vi "Camera_Read and Save Settings.vi"(8 "Error":errorcluster, 10 "CameraDevRef":T7, 11 "Camera Address":string) -> (0 "Error Out":errorcluster, 1 "Output Cluster Out":T1, 2 "Camera Settings Out":T2 {"Saturation" min=0 max=100 step=1; "Sharpness" min=0 max=100 step=1; "Brightness" min=0 max=100 step=1; "Exposure (%)" min=0.0 max=100.0 step=1.0}, 3 "CameraDevRef Out":T7)   [LabVIEW 2017, in "VisionSystem.lvlib"]
uses:
  VisionSystem.lvlib
  <vilib>/Rock Robotics/WPI/Camera/WPI_CameraDevRef.ctl
  TypeDefs/Cluster_Camera Settings.ctl
  <vilib>/Rock Robotics/WPI/Camera/WPI_CameraImageSize.ctl
  <vilib>/Rock Robotics/WPI/Camera/WPI_CameraFrameRate.ctl
  <vilib>/Rock Robotics/WPI/Camera/WPI_CameraWhite Balance Values.ctl
  <vilib>/Rock Robotics/WPI/Camera/WPI_CameraExposure Values.ctl
  <vilib>/Rock Robotics/WPI/Camera/WPI_CameraSettings Control.ctl
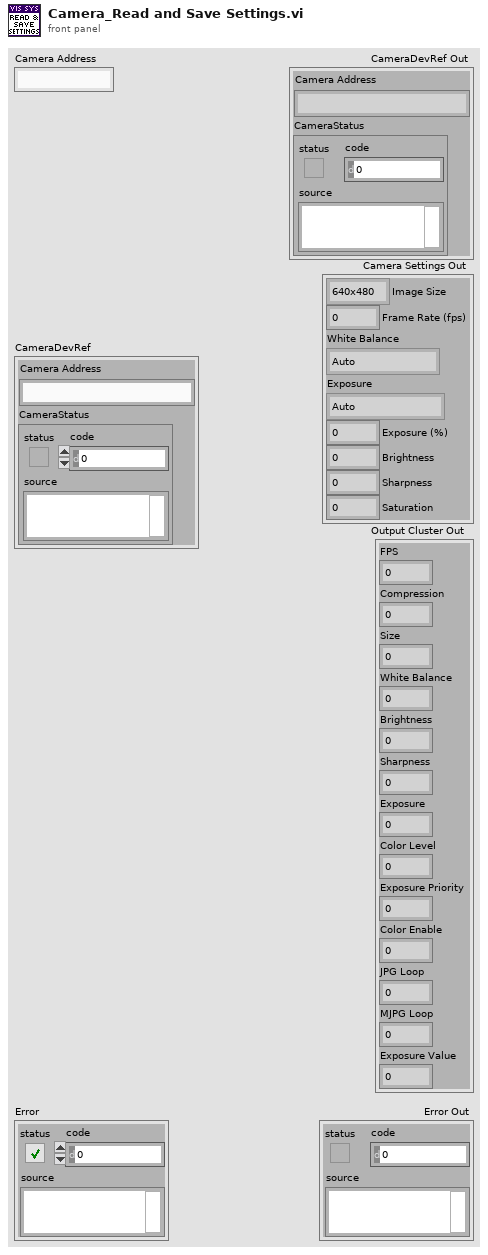
[diagram p1: front panel]
types:
  T1 = typedef "WPI_CameraSettings Control.ctl" = cluster{"FPS":i32, "Compression":i32, "Size":i32, "White Balance":i32, "Brightness":i32, "Sharpness":i32, "Exposure":i32, "Color Level":i32, "Exposure Priority":i32, "Color Enable":i32, "JPG Loop":i32, "MJPG Loop":i32, "Exposure Value":i32}
  T2 = typedef "Cluster_Camera Settings.ctl" = cluster{"Image Size":T3, "Frame Rate (fps)":T4, "White Balance":T5, "Exposure":T6, "Exposure (%)":dbl, "Brightness":i32, "Sharpness":i32, "Saturation":i32}
  T3 = typedef "WPI_CameraImageSize.ctl" = enum16{"640x480", "320x240", "160x120", "Custom"}
  T4 = typedef "WPI_CameraFrameRate.ctl" = u32
  T5 = typedef "WPI_CameraWhite Balance Values.ctl" = enum16{"Auto", "Fixed indoor", "Fixed outdoor 1", "Fixed outdoor 2", "Fixed fluorescent 1", "Fixed fluorescent 2", "Hold current", "Custom"}
  T6 = typedef "WPI_CameraExposure Values.ctl" = enum16{"Auto", "Flicker-free 50 Hz", "Flicker-free 60 Hz", "Hold current", "Custom"}
  T7 = typedef "WPI_CameraDevRef.ctl" = cluster{"Camera Address":string, "CameraStatus":errorcluster}
  T8 = typedef "WPI_CameraExposure Priority Values.ctl" = enum16{"None", "Prioritize frame rate", "Prioritize image quality"}
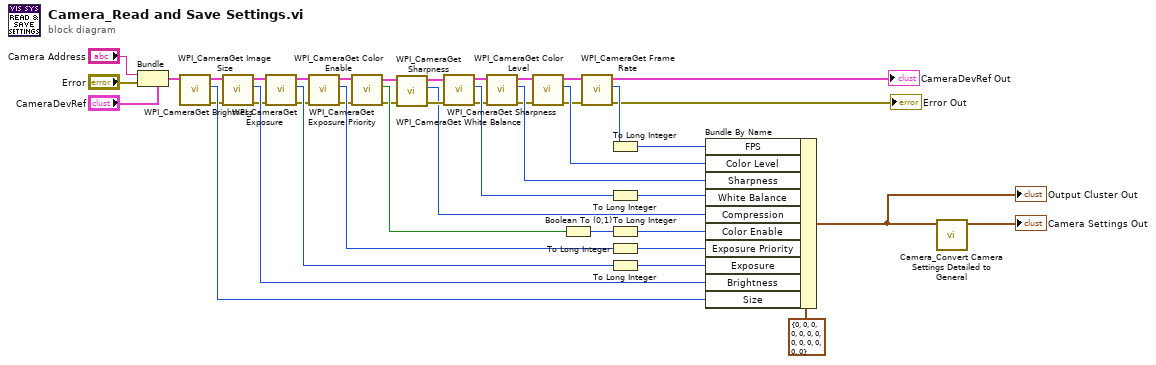
[diagram p0: block diagram]
diagram:
  n1 = Bundle(cluster="CameraDevRef", "Camera Address"="Camera Address", "CameraStatus"="Error") -> (w43:T7)
  n2 = call <vilib>:"WPI_CameraGet Image Size.vi"("CameraDevRef"=w43) -> ("error out"=w15:errorcluster, "Image Size"=w25:T3, "CameraDevRef Out"=w37:T7)  [unwired: 7 in, 1 out]
  n3 = call <vilib>:"WPI_CameraGet Brightness.vi"("error in (no error)"=w15, "CameraDevRef"=w37) -> ("error out"=w14:errorcluster, "Brightness"=w26:i32, "CameraDevRef Out"=w38:T7)  [unwired: 7 in]
  n4 = call <vilib>:"WPI_CameraGet Exposure.vi"("error in (no error)"=w14, "CameraDevRef"=w38) -> ("error out"=w13:errorcluster, "Exposure"=w27:T6, "CameraDevRef Out"=w39:T7)  [unwired: 6 in, 1 out]
  n5 = call <vilib>:"WPI_CameraGet Exposure Priority.vi"("error in (no error)"=w13, "CameraDevRef"=w39) -> ("error out"=w12:errorcluster, "Exposure Priority"=w28:T8, "CameraDevRef Out"=w40:T7)  [unwired: 7 in]
  n6 = call <vilib>:"WPI_CameraGet Color Enable.vi"("error in (no error)"=w12, "CameraDevRef"=w40) -> ("error out"=w5:errorcluster, "Color Enabled"=w35:bool, "CameraDevRef Out"=w2:T7)  [unwired: 7 in]
  n7 = call <vilib>:"WPI_CameraGet Sharpness.vi"("error in (no error)"=w5, "CameraDevRef"=w2) -> ("error out"=w4:errorcluster, "Sharpness"=w1:i32, "CameraDevRef Out"=w3:T7)  [unwired: 7 in]
  n8 = call <vilib>:"WPI_CameraGet White Balance.vi"("error in (no error)"=w4, "CameraDevRef"=w3) -> ("error out"=w11:errorcluster, "White Balance"=w20:T5, "CameraDevRef Out"=w42:T7)  [unwired: 6 in, 1 out]
  n9 = call <vilib>:"WPI_CameraGet Sharpness.vi"("error in (no error)"=w11, "CameraDevRef"=w42) -> ("error out"=w10:errorcluster, "Sharpness"=w30:i32, "CameraDevRef Out"=w41:T7)  [unwired: 7 in]
  n10 = call <vilib>:"WPI_CameraGet Color Level.vi"("error in (no error)"=w10, "CameraDevRef"=w41) -> ("error out"=w9:errorcluster, "Color Level"=w31:i32, "CameraDevRef Out"=w24:T7)  [unwired: 7 in]
  n11 = Boolean To (0,1)(Boolean=w35) -> (0, 1=w29:i16)
  n12 = call <vilib>:"WPI_CameraGet Frame Rate.vi"("error in (no error)"=w9, "CameraDevRef"=w24) -> ("error out"=→"Error Out":errorcluster, "Frame Rate (fps)"=w22:T4, "CameraDevRef Out"=→"CameraDevRef Out":T7)  [unwired: 7 in]
  n13 = To Long Integer(number=w22) -> (32bit integer=w21:i32)
  n14 = To Long Integer(number=w20) -> (32bit integer=w19:i32)
  n15 = To Long Integer(number=w29) -> (32bit integer=w18:i32)
  n16 = To Long Integer(number=w28) -> (32bit integer=w17:i32)
  n17 = To Long Integer(number=w27) -> (32bit integer=w16:i32)
  n18 = Bundle By Name(cluster=T1 {"FPS"=0, "Compression"=0, "Size"=0, "White Balance"=0, "Brightness"=0, "Sharpness"=0, "Exposure"=0, "Color Level"=0, "Exposure Priority"=0, "Color Enable"=0, "JPG Loop"=0, "MJPG Loop"=0, "Exposure Value"=0} ("Values In"), "FPS"=w21, "Color Level"=w31, "Sharpness"=w30, "White Balance"=w19, "Compression"=w1, "Color Enable"=w18, "Exposure Priority"=w17, "Exposure"=w16, "Brightness"=w26, "Size"=w25) -> (w6:T1)
  "Output Cluster Out" <- w6
  n19 = call "Camera_Convert Camera Settings Detailed to General .vi"("Values"=w6) -> ("Camera Settings"=→"Camera Settings Out":T2)  [unwired: 9 in, 1 out]
